vi "testing_query_settings.vi"() -> ()   [LabVIEW 2015, in "Tausand AB1000.lvlib"]
uses:
  <instrlib>/Tausand AB1000/Tausand AB1000.lvlib
  <instrlib>/Tausand AB1000/Public/Controls/deviceTypeRing.ctl
  <instrlib>/Tausand AB1000/Public/Controls/channelRing.ctl
  <instrlib>/Tausand AB1000/Public/Controls/configMultipleCoincRing.ctl
panel:
  out "device type Q?":T1 items=["any"=0, "AB1002"=1002, "AB1004"=1004, "AB1502"=1502, "AB1504"=1504, "AB2002"=2002, "AB2004"=2004, "AB2502"=2502, "AB2504"=2504]
  in  "VISA resource name":refnum<visa-resource-name>
  in  "error in (no error)":errorcluster
  out "error out":errorcluster
  out "all checksum ok?":bool
  out "all labels":string[](array[string])
  out "all values":u32[](array[numeric])
  in  "read timeout (500 ms)":u32=500
  in  "device type allstg":T1 items=["any"=0, "AB1002"=1002, "AB1004"=1004, "AB1502"=1502, "AB1504"=1504, "AB2002"=2002, "AB2004"=2004, "AB2502"=2502, "AB2504"=2504]
  out "cw checksum ok?":bool
  out "cw value ns":u32
  in  "device type cw":T1 items=["any"=0, "AB1002"=1002, "AB1004"=1004, "AB1502"=1502, "AB1504"=1504, "AB2002"=2002, "AB2004"=2004, "AB2502"=2502, "AB2504"=2504]
  out "del checksum ok?":bool
  out "del value ns":u32
  in  "channel del":T2 items=["none", "A", "B", "C", "D", "E", "F", "G", "H"]
  in  "device type del":T1 items=["any"=0, "AB1002"=1002, "AB1004"=1004, "AB1502"=1502, "AB1504"=1504, "AB2002"=2002, "AB2004"=2004, "AB2502"=2502, "AB2504"=2504]
  out "mc checksum ok?":bool
  out "multi-fold channels []":T3[](array[typedef]) items=["ABC"=224, "ABD"=208, "ABE"=200, "ABF"=196, "ABG"=194, "ABH"=193, "ACD"=176, "ACE"=168, "ACF"=164, "ACG"=162, "ACH"=161, "ADE"=152, "ADF"=148, "ADG"=146, "ADH"=145, "AEF"=140, "AEG"=138, "AEH"=137, "AFG"=134, "AFH"=133, "AGH"=131, "BCD"=112, "BCE"=104, "BCF"=100, "BCG"=98, "BCH"=97, "BDE"=88, "BDF"=84, "BDG"=82, "BDH"=81, "BEF"=76, "BEG"=74, "BEH"=73, "BFG"=70, "BFH"=69, "BGH"=67, "CDE"=56, "CDF"=52, "CDG"=50, "CDH"=49, "CEF"=44, "CEG"=42, "CEH"=41, "CFG"=38, "CFH"=37, "CGH"=35, "DEF"=28, "DEG"=26, "DEH"=25, "DFG"=22, "DFH"=21, "DGH"=19, "EFG"=14, "EFH"=13, "EGH"=11, "FGH"=7, "ABCD"=240, "ABCE"=232, "ABCF"=228, "ABCG"=226, "ABCH"=225, "ABDE"=216, "ABDF"=212, "ABDG"=210, "ABDH"=209, "ABEF"=204, "ABEG"=202, "ABEH"=201, "ABFG"=198, "ABFH"=197, "ABGH"=195, "ACDE"=184, "ACDF"=180, "ACDG"=178, "ACDH"=177, "ACEF"=172, "ACEG"=170, "ACEH"=169, "ACFG"=166, "ACFH"=165, "ACGH"=163, "ADEF"=156, "ADEG"=154, "ADEH"=153, "ADFG"=150, "ADFH"=149, "ADGH"=147, "AEFG"=142, "AEFH"=141, "AEGH"=139, "AFGH"=135, "BCDE"=120, "BCDF"=116, "BCDG"=114, "BCDH"=113, "BCEF"=108, "BCEG"=106, "BCEH"=105, "BCFG"=102, "BCFH"=101, "BCGH"=99, "BDEF"=92, "BDEG"=90, "BDEH"=89, "BDFG"=86, "BDFH"=85, "BDGH"=83, "BEFG"=78, "BEFH"=77, "BEGH"=75, "BFGH"=71, "CDEF"=60, "CDEG"=58, "CDEH"=57, "CDFG"=54, "CDFH"=53, "CDGH"=51, "CEFG"=46, "CEFH"=45, "CEGH"=43, "CFGH"=39, "DEFG"=30, "DEFH"=29, "DEGH"=27, "DFGH"=23, "EFGH"=15]
  in  "device type mc":T1 items=["any"=0, "AB1002"=1002, "AB1004"=1004, "AB1502"=1502, "AB1504"=1504, "AB2002"=2002, "AB2004"=2004, "AB2502"=2502, "AB2504"=2504]
  out "smp checksum ok?":bool
  out "smp value ms":u32
  in  "device type smp":T1 items=["any"=0, "AB1002"=1002, "AB1004"=1004, "AB1502"=1502, "AB1504"=1504, "AB2002"=2002, "AB2004"=2004, "AB2502"=2502, "AB2504"=2504]
  out "slp checksum ok?":bool
  out "slp value ns":u32
  in  "channel sl":T2 items=["none", "A", "B", "C", "D", "E", "F", "G", "H"]
  in  "device type slp":T1 items=["any"=0, "AB1002"=1002, "AB1004"=1004, "AB1502"=1502, "AB1504"=1504, "AB2002"=2002, "AB2004"=2004, "AB2502"=2502, "AB2504"=2504]
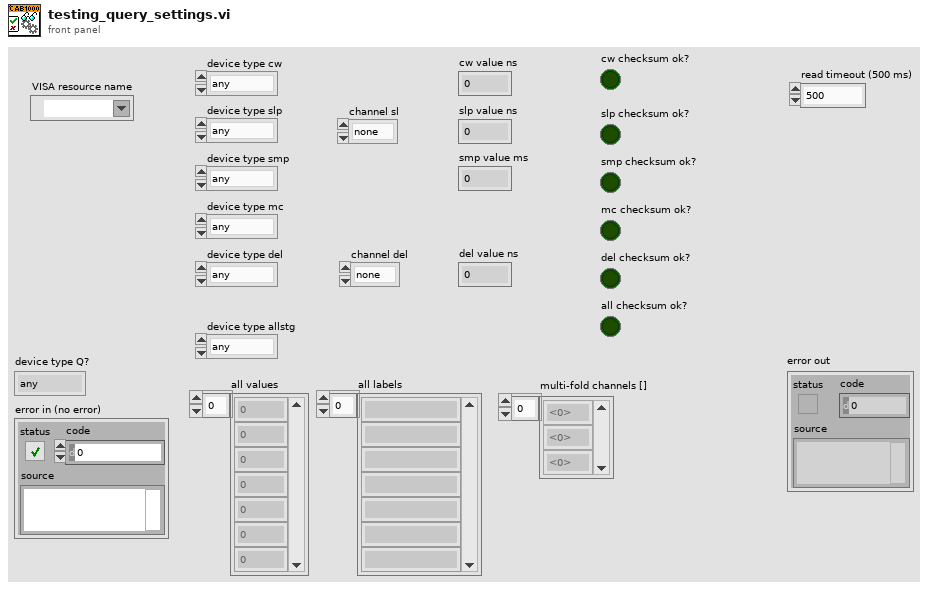
[diagram p1: front panel]
types:
  T1 = typedef "Tausand AB1000.lvlib/deviceTypeRing.ctl" = u16
  T2 = typedef "Tausand AB1000.lvlib/channelRing.ctl" = u8
  T3 = typedef "Tausand AB1000.lvlib/configMultipleCoincRing.ctl" = u16
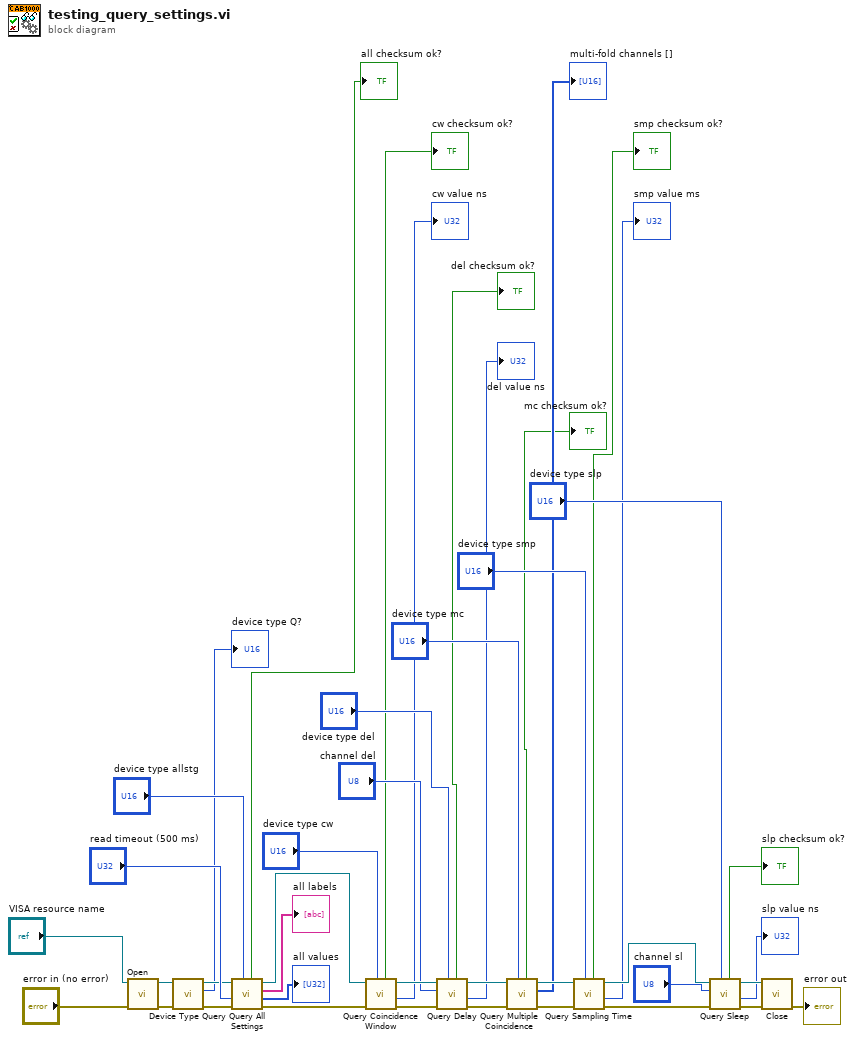
[diagram p0: block diagram]
diagram:
  n1 = call <instrlib>:"Open.vi"("error in (no error)"="error in (no error)", "VISA resource name"="VISA resource name") -> ("error out"=w4:errorcluster, "VISA resource name out"=w5:refnum<visa-resource-name>)  [unwired: 8 in]
  n2 = call <instrlib>:"Device Type Query.vi"("error in (no error)"=w4, "VISA Refnum in"=w5) -> ("error out"=w3:errorcluster, "device type"=→"device type Q?":T1, "VISA Refnum out"=w2:refnum<visa-resource-name>)  [unwired: 7 in]
  n3 = call <instrlib>:"Query All Settings.vi"("device type"="device type allstg", "error in (no error)"=w3, "read timeout (500 ms)"="read timeout (500 ms)", "VISA Refnum in"=w2) -> ("error out"=w41:errorcluster, "values"=→"all values":u32[], "labels"=→"all labels":string[], "VISA Refnum out"=w42:refnum<visa-resource-name>, "checksum ok?"=→"all checksum ok?":bool)  [unwired: 3 in]
  n4 = call <instrlib>:"Query Coincidence Window.vi"("device type"="device type cw", "error in (no error)"=w41, "VISA Refnum in"=w42) -> ("error out"=w40:errorcluster, "value ns out"=→"cw value ns":u32, "VISA Refnum out"=w31:refnum<visa-resource-name>, "checksum ok?"=→"cw checksum ok?":bool)  [unwired: 5 in]
  n5 = call <instrlib>:"Query Delay.vi"("device type"="device type del", "error in (no error)"=w40, "channel"="channel del", "VISA Refnum in"=w31) -> ("error out"=w39:errorcluster, "value ns out"=→"del value ns":u32, "VISA Refnum out"=w32:refnum<visa-resource-name>, "checksum ok?"=→"del checksum ok?":bool)  [unwired: 4 in]
  n6 = call <instrlib>:"Query Multiple Coincidence.vi"("device type"="device type mc", "error in (no error)"=w39, "VISA Refnum in"=w32) -> ("error out"=w38:errorcluster, "multi-fold channels []"=→"multi-fold channels []":T3[], "VISA Refnum out"=w33:refnum<visa-resource-name>, "checksum ok?"=→"mc checksum ok?":bool)  [unwired: 5 in]
  n7 = call <instrlib>:"Query Sampling Time.vi"("device type"="device type smp", "error in (no error)"=w38, "VISA Refnum in"=w33) -> ("error out"=w37:errorcluster, "value ms out"=→"smp value ms":u32, "VISA Refnum out"=w34:refnum<visa-resource-name>, "checksum ok?"=→"smp checksum ok?":bool)  [unwired: 5 in]
  n8 = call <instrlib>:"Query Sleep.vi"("device type"="device type slp", "error in (no error)"=w37, "channel"="channel sl", "VISA Refnum in"=w34) -> ("error out"=w36:errorcluster, "value ns out"=→"slp value ns":u32, "VISA Refnum out"=w35:refnum<visa-resource-name>, "checksum ok?"=→"slp checksum ok?":bool)  [unwired: 4 in]
  n9 = call <instrlib>:"Close.vi"("error in (no error)"=w36, "VISA resource name"=w35) -> ("error out"=→"error out":errorcluster)  [unwired: 9 in]
